vi "Do.vi"(8 "error in (no error)":errorcluster, 10 "Actor in":refnum<class "Actor.lvclass">, 11 "Response Msg":refnum<class "Response Msg.lvclass">) -> (0 "error out":errorcluster, 2 "Actor out":refnum<class "Actor.lvclass">)   [LabVIEW 2020, in "Publisher.lvlib" / "Response Msg.lvclass"]
doc: "This Do implementation will execute Core and then Respond on Data and lastly Publish Data if this is not handled on the sender."
uses:
  Response Msg.lvclass
  PPL/HDH.Actor Framework.Core.Actor.lvlibp/1abvi3w/vi.lib/ActorFramework/Actor/Actor.lvclass
  Response Msg.lvclass/Response Msg.ctl
  PPL/HDH.Actor Framework.Core.Actor.lvlibp/1abvi3w/vi.lib/ActorFramework/Message Enqueuer/Message Priority.ctl
  Response Core/Response Core/Response Core.lvclass
  PPL/HDH.Actor Framework.Core.Actor.lvlibp/1abvi3w/vi.lib/ActorFramework/Message Enqueuer/Message Enqueuer.lvclass
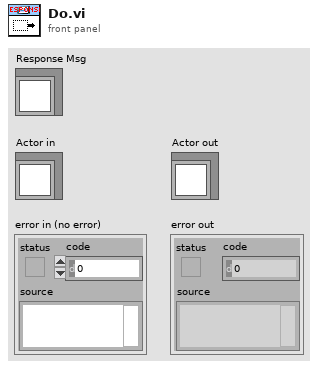
[diagram p1: front panel]
types:
  T1 = typedef "HDH.Actor Framework.Core.Actor.lvlibp/Message Enqueuer.lvclass/Message Priority.ctl" = enum16{"Low", "Normal", "High"}
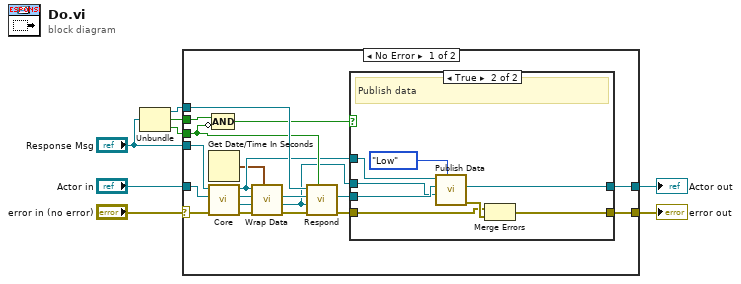
[diagram p0: block diagram]
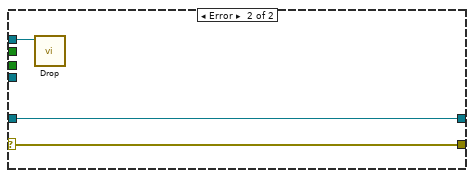
[diagram p3: hidden frame]
diagram:
  n1 = Unbundle("Response Msg") -> (w3:refnum<class "Response Core.lvclass">, w1:bool, w2:bool)
  n2 = case shown="No Error" "error in (no error)" {
    selector: "error in (no error)" -> [w26 w40]
    tunnel: [w21 w40] -> w8
    tunnel: "Actor in" -> [w11 w38]
    tunnel: "Response Msg" -> [w27 _]
    tunnel: [w23 w38] -> w5
    tunnel: w3 -> [w25 w39]
    tunnel: w2 -> [w19 _]
    tunnel: w1 -> [w20 _]
    frame No Error {
      n3 = Get Date/Time In Seconds() -> (seconds since 1Jan1904=w12:timestamp)
      n4 = call-dynamic "Core.vi"("error in (no error)"=w26, "Actor in"=w11, "Response Msg in"=w27) -> ("error out"=w14:errorcluster, "Data"=w9:refnum<class "Data.lvclass">, "Actor out"=w10:refnum<class "Actor.lvclass">, "Response Msg out"=w17:refnum<class "Response Msg.lvclass">)  [unwired: 5 in]
      n5 = Compound Arithmetic op=AND(w20, invert w19) -> (w18:bool)
      n6 = call-dynamic "Wrap Data.vi"("Start Time"=w12, "error in (no error)"=w14, "Data in"=w9, "Actor in"=w10, "Response Msg"=w17) -> ("error out"=w13:errorcluster, "Data out"=w15:refnum<class "Data.lvclass">, "Actor out"=w16:refnum<class "Actor.lvclass">)  [unwired: 4 in]
      n7 = call-dynamic "Respond.vi"("Sender is Waiting?(F)"=w19, "error in (no error)"=w13, "Data"=w15, "Actor in"=w16, "Response Core in"=w25) -> ("error out"=w22:errorcluster, "Actor out"=w24:refnum<class "Actor.lvclass">)  [unwired: 5 in]
      n8 = case shown="True" w18 {
        tunnel: w22 -> [w29 w32]
        tunnel: [w29 w33] -> w21
        tunnel: [w28 w36] -> w23
        tunnel: w24 -> [w28 w35]
        tunnel: w17 -> [_ w34]
        tunnel: w15 -> [_ w30]
        frame False {
          # "'Do not publish' or 'Handled on the sender'"
        }
        frame True {
          # "Publish data"
          n9 = call-dynamic "Publish Data.vi"("Message Priority (Normal)"=Message_Priority."Low", "Data"=w30, "Actor in"=w35, "Response Msg"=w34) -> ("error out"=w37:errorcluster, "Actor out"=w36:refnum<class "Actor.lvclass">)  [unwired: 6 in]
          n10 = Merge Errors(w32, w37) -> (w33:errorcluster)
        }
      }
    }
    frame Error {
      n11 = call-dynamic "Drop.vi"("Response Core in"=w39) -> ()  [unwired: 11 in]
    }
  }
  "error out" <- w8
  "Actor out" <- w5
